vi "createPlatformData.vi"() -> (1 "platforms to \nlower":i32[](array[numeric]), 3 "platforms to \nraise":i32[](array[numeric]))   [LabVIEW 2017]
panel:
  in  "Platform 61":bool
  in  "Platform 60":bool
  in  "Platform 59":bool
  in  "Platform 58":bool
  in  "Platform 57":bool
  in  "Platform 56":bool
  in  "Platform 55":bool
  in  "Platform 54":bool
  in  "Platform 53":bool
  in  "Platform 52":bool
  in  "Platform 51":bool
  in  "Platform 50":bool
  in  "Platform 49":bool
  in  "Platform 48":bool
  in  "Platform 47":bool
  in  "Platform 46":bool
  in  "Platform 45":bool
  in  "Platform 44":bool
  in  "Platform 43":bool
  in  "Platform 42":bool
  in  "Platform 41":bool
  in  "Platform 40":bool
  in  "Platform 39":bool
  in  "Platform 38":bool
  in  "Platform 37":bool
  in  "Platform 36":bool
  in  "Platform 35":bool
  in  "Platform 34":bool
  in  "Platform 33":bool
  in  "Platform 32":bool
  in  "Platform 31":bool
  in  "Platform 30":bool
  in  "Platform 29":bool
  in  "Platform 28":bool
  in  "Platform 27":bool
  in  "Platform 26":bool
  in  "Platform 25":bool
  in  "Platform 24":bool
  in  "Platform 23":bool
  in  "Platform 22":bool
  in  "Platform 21":bool
  in  "Platform 20":bool
  in  "Platform 19":bool
  in  "Platform 18":bool
  in  "Platform 17":bool
  in  "Platform 16":bool
  in  "Platform 15":bool
  in  "Platform 14":bool
  in  "Platform 13":bool
  in  "Platform 12":bool
  in  "Platform 11":bool
  in  "Platform 10":bool
  in  "Platform 9":bool
  in  "Platform 8":bool
  in  "Platform 7":bool
  in  "Platform 6":bool
  in  "Platform 5":bool
  in  "Platform 4":bool
  in  "Platform 3":bool
  in  "Platform 2":bool
  in  "Platform 1":bool
  in  "Select?":bool
  in  "Platform 61":bool
  in  "Platform 60":bool
  in  "Platform 59":bool
  in  "Platform 58":bool
  in  "Platform 57":bool
  in  "Platform 56":bool
  in  "Platform 55":bool
  in  "Platform 54":bool
  in  "Platform 53":bool
  in  "Platform 52":bool
  in  "Platform 51":bool
  in  "Platform 50":bool
  in  "Platform 49":bool
  in  "Platform 48":bool
  in  "Platform 47":bool
  in  "Platform 46":bool
  in  "Platform 45":bool
  in  "Platform 44":bool
  in  "Platform 43":bool
  in  "Platform 42":bool
  in  "Platform 41":bool
  in  "Platform 40":bool
  in  "Platform 39":bool
  in  "Platform 38":bool
  in  "Platform 37":bool
  in  "Platform 36":bool
  in  "Platform 35":bool
  in  "Platform 34":bool
  in  "Platform 33":bool
  in  "Platform 32":bool
  in  "Platform 31":bool
  in  "Platform 30":bool
  in  "Platform 29":bool
  in  "Platform 28":bool
  in  "Platform 27":bool
  in  "Platform 26":bool
  in  "Platform 25":bool
  in  "Platform 24":bool
  in  "Platform 23":bool
  in  "Platform 22":bool
  in  "Platform 21":bool
  in  "Platform 20":bool
  in  "Platform 19":bool
  in  "Platform 18":bool
  in  "Platform 17":bool
  in  "Platform 16":bool
  in  "Platform 15":bool
  in  "Platform 14":bool
  in  "Platform 13":bool
  in  "Platform 12":bool
  in  "Platform 11":bool
  in  "Platform 10":bool
  in  "Platform 9":bool
  in  "Platform 8":bool
  in  "Platform 7":bool
  in  "Platform 6":bool
  in  "Platform 5":bool
  in  "Platform 4":bool
  in  "Platform 3":bool
  in  "Platform 2":bool
  in  "Platform 1":bool
  # "Platforms up"
  # "Platforms down"
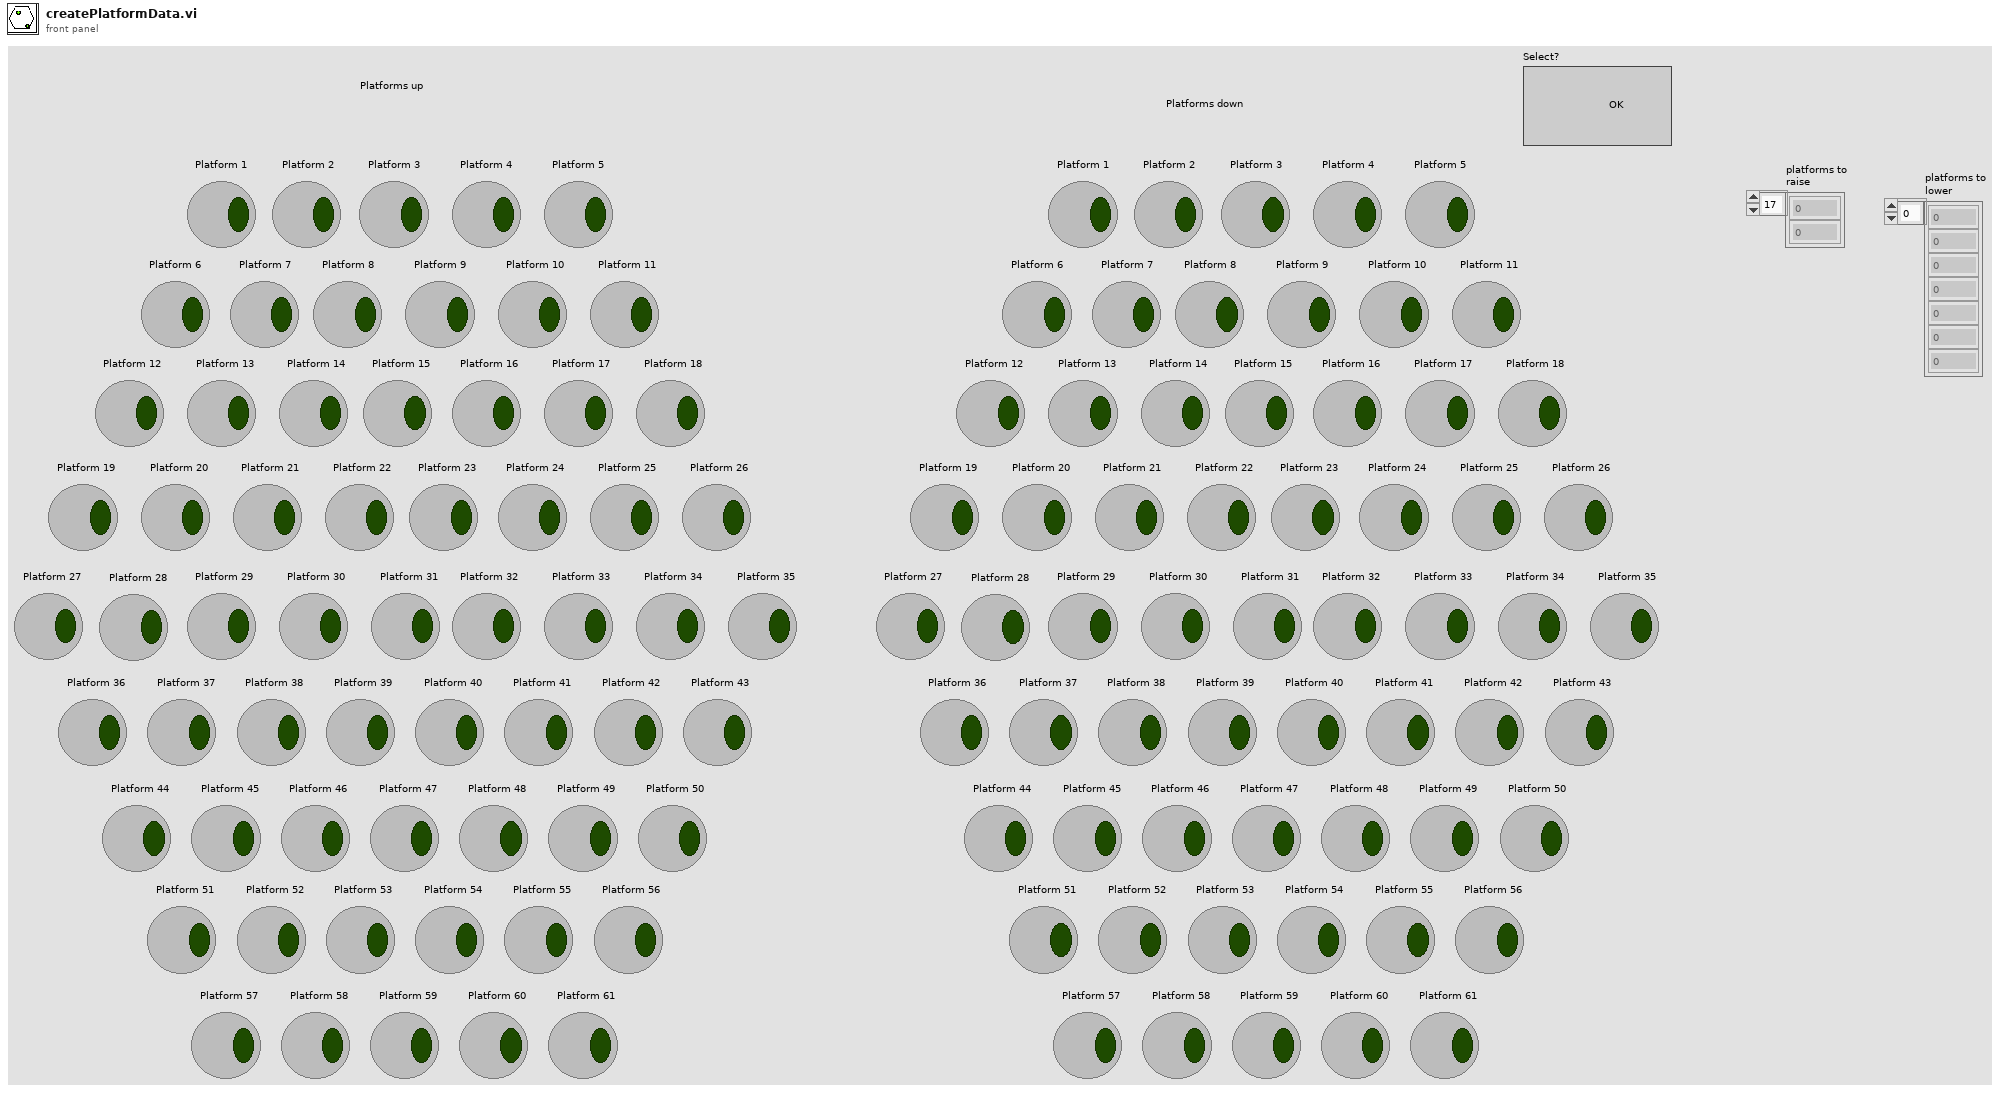
[diagram p1: front panel]
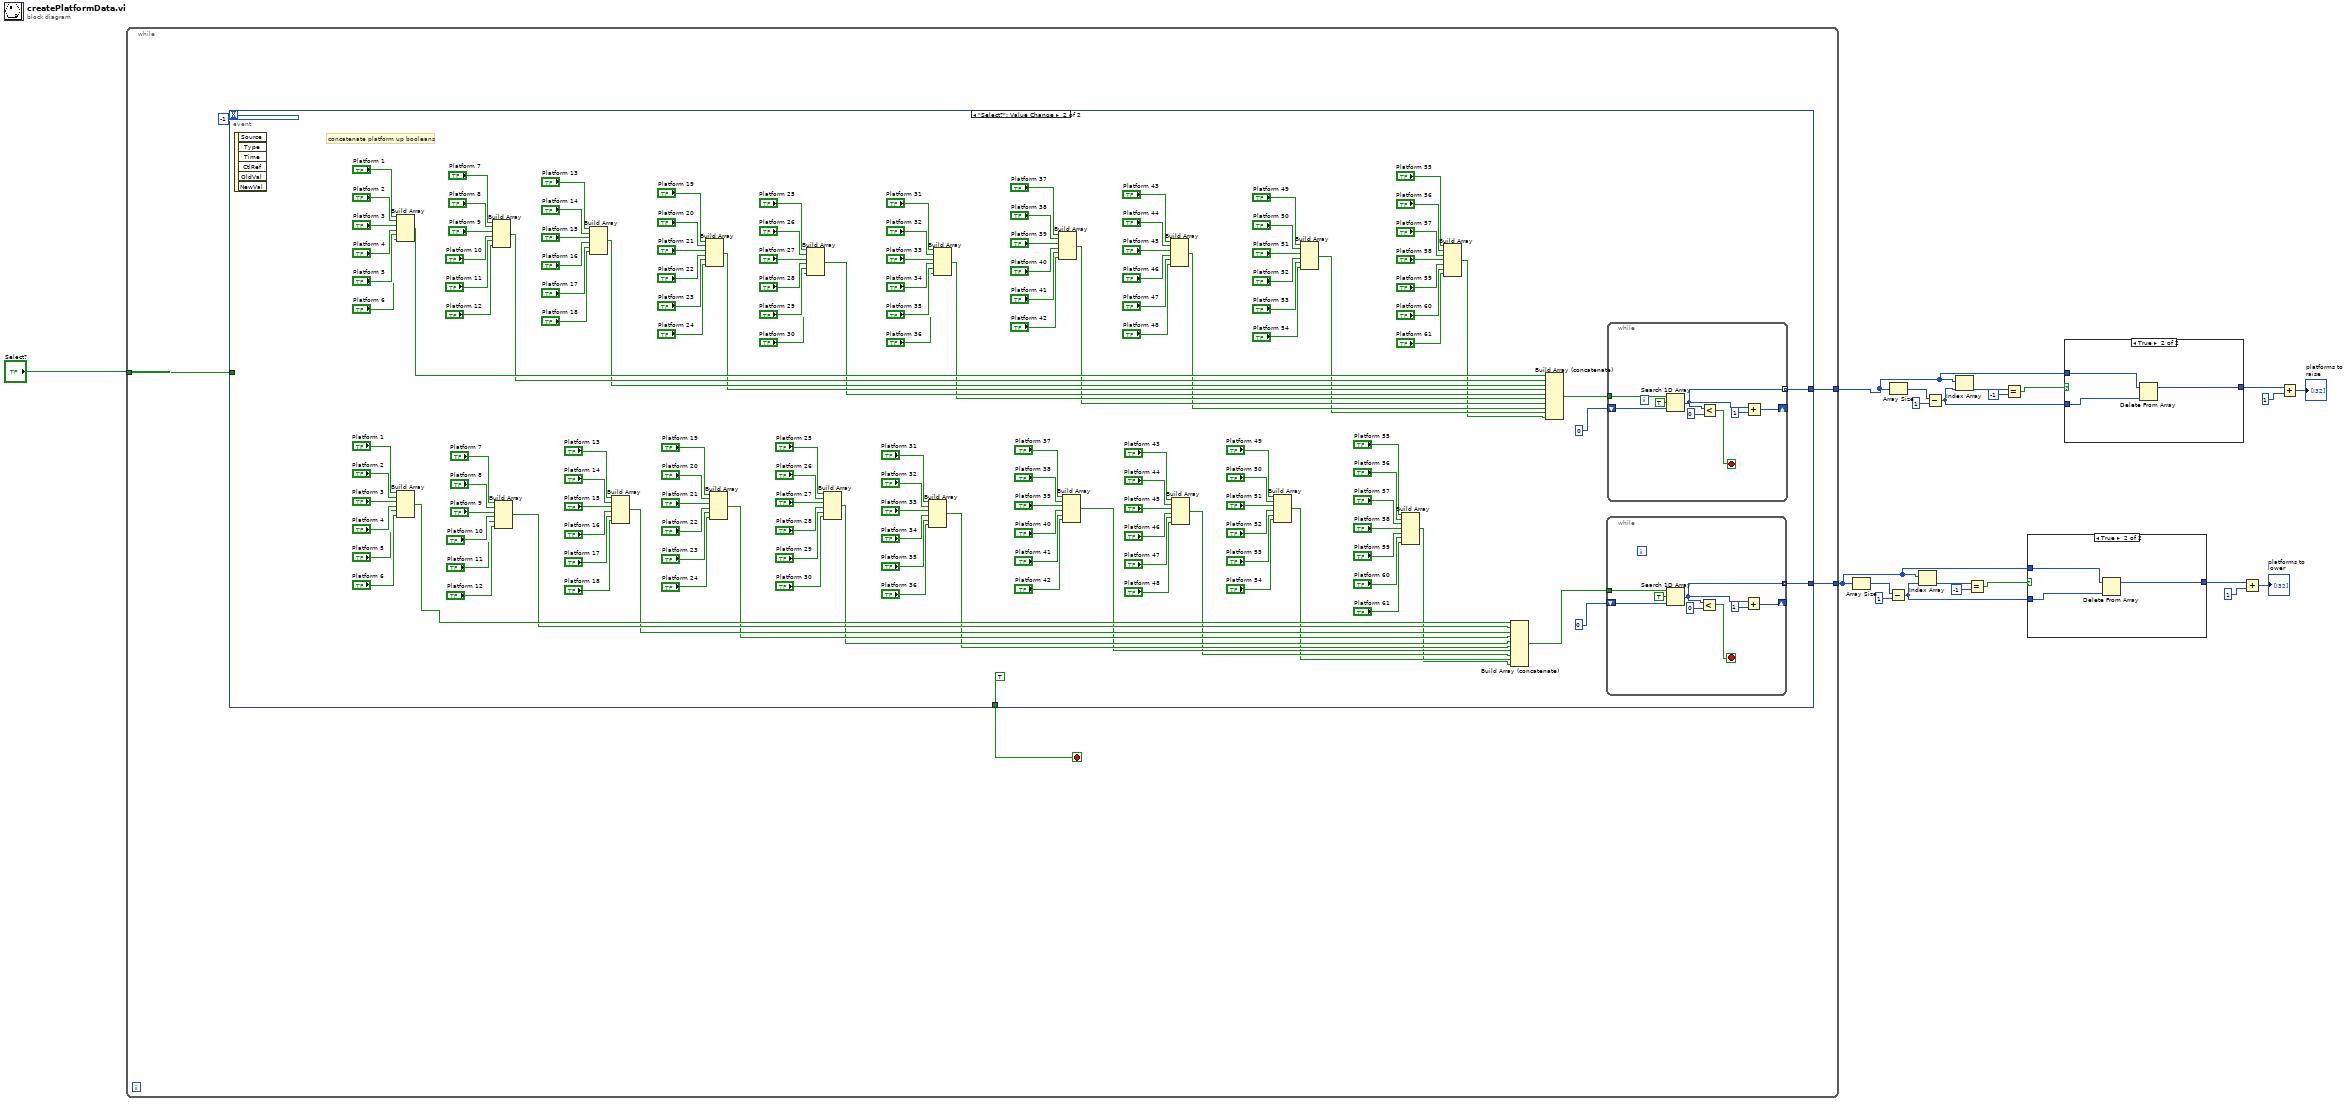
[diagram p0: block diagram]
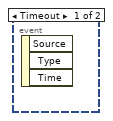
[diagram p4: hidden frame]
diagram:
  n1 = while {
    tunnel: "Select?" -> [w25]
    tunnel: [w23] -> w1
    tunnel: [w22] -> w17
    stop <- w24 stop-if-true
    n2 = event shown="[1] \"Select?\": Value Change" {
      selector: _ -> [_ _]
      dyn-events: _ -> [_ _]
      timeout: -1 -> [_ _]
      tunnel: w25 -> [_ _]
      tunnel: [_ TRUE] -> w24
      tunnel: [_ w41] -> w23
      tunnel: [_ w27] -> w22
      event Timeout {
        n3 = event-data() -> ()  [unwired: 1 in, 3 out]
      }
      event "Select?": Value Change {
        # "concatenate platform up booleans"
        n4 = event-data() -> ()  [unwired: 1 in, 6 out]
        n5 = Build Array("Platform 1", "Platform 2", "Platform 3", "Platform 4", "Platform 5", "Platform 6") -> (w39:bool[])
        n6 = Build Array("Platform 1", "Platform 2", "Platform 3", "Platform 4", "Platform 5", "Platform 6") -> (w53:bool[])
        n7 = Build Array("Platform 7", "Platform 8", "Platform 9", "Platform 10", "Platform 11", "Platform 12") -> (w52:bool[])
        n8 = Build Array("Platform 7", "Platform 8", "Platform 9", "Platform 10", "Platform 11", "Platform 12") -> (w38:bool[])
        n9 = Build Array("Platform 13", "Platform 14", "Platform 15", "Platform 16", "Platform 17", "Platform 18") -> (w51:bool[])
        n10 = Build Array("Platform 13", "Platform 14", "Platform 15", "Platform 16", "Platform 17", "Platform 18") -> (w37:bool[])
        n11 = Build Array("Platform 19", "Platform 20", "Platform 21", "Platform 22", "Platform 23", "Platform 24") -> (w50:bool[])
        n12 = Build Array("Platform 19", "Platform 20", "Platform 21", "Platform 22", "Platform 23", "Platform 24") -> (w36:bool[])
        n13 = Build Array("Platform 25", "Platform 26", "Platform 27", "Platform 28", "Platform 29", "Platform 30") -> (w49:bool[])
        n14 = Build Array("Platform 25", "Platform 26", "Platform 27", "Platform 28", "Platform 29", "Platform 30") -> (w35:bool[])
        n15 = Build Array("Platform 31", "Platform 32", "Platform 33", "Platform 34", "Platform 35", "Platform 36") -> (w34:bool[])
        n16 = Build Array("Platform 31", "Platform 32", "Platform 33", "Platform 34", "Platform 35", "Platform 36") -> (w48:bool[])
        n17 = Build Array("Platform 37", "Platform 38", "Platform 39", "Platform 40", "Platform 41", "Platform 42") -> (w47:bool[])
        n18 = Build Array("Platform 37", "Platform 38", "Platform 39", "Platform 40", "Platform 41", "Platform 42") -> (w33:bool[])
        n19 = Build Array("Platform 43", "Platform 44", "Platform 45", "Platform 46", "Platform 47", "Platform 48") -> (w46:bool[])
        n20 = Build Array("Platform 43", "Platform 44", "Platform 45", "Platform 46", "Platform 47", "Platform 48") -> (w32:bool[])
        n21 = Build Array("Platform 49", "Platform 50", "Platform 51", "Platform 52", "Platform 53", "Platform 54") -> (w31:bool[])
        n22 = Build Array("Platform 49", "Platform 50", "Platform 51", "Platform 52", "Platform 53", "Platform 54") -> (w45:bool[])
        n23 = Build Array("Platform 55", "Platform 56", "Platform 57", "Platform 58", "Platform 59", "Platform 60", "Platform 61") -> (w30:bool[])
        n24 = Build Array("Platform 55", "Platform 56", "Platform 57", "Platform 58", "Platform 59", "Platform 60", "Platform 61") -> (w44:bool[])
        n25 = Build Array (concatenate)(w39, w38, w37, w36, w35, w34, w33, w32, w31, w30) -> (w28:bool[])
        n26 = Build Array (concatenate)(w53, w52, w51, w50, w49, w48, w47, w46, w45, w44) -> (w43:bool[])
        n27 = while {
          tunnel: w28 -> [w176]
          shift-right: [w178] -> _
          shift-left: 0 ("start index (0)") -> [w182]
          tunnel: [w179] -> w27 mode=indexing
          stop <- w180 stop-if-true
          n28 = Search 1D Array(1D array=w176, element=TRUE, start index (0)=w182) -> (index of element=w179:i32)
          n29 = Less?(x=w179, y=0) -> (x < y?=w180:bool)
          n30 = Add(x=w179, y=1) -> (x+y=w178:i32)
        }
        n31 = while {
          tunnel: w43 -> [w191]
          shift-right: [w185] -> _
          shift-left: 0 ("start index (0)") -> [w189]
          tunnel: [w186] -> w41 mode=indexing
          stop <- w187 stop-if-true
          n32 = Search 1D Array(1D array=w191, element=TRUE, start index (0)=w189) -> (index of element=w186:i32)
          n33 = Less?(x=w186, y=0) -> (x < y?=w187:bool)
          n34 = Add(x=w186, y=1) -> (x+y=w185:i32)
        }
      }
    }
  }
  n35 = Array Size(array=w17) -> (size(s)=w15:i32)
  n36 = Subtract(x=w15, y=1) -> (x-y=w14:i32)
  n37 = Array Size(array=w1) -> (size(s)=w6:i32)
  n38 = Index Array(array=w17, index=w14) -> (element=w20:i32)
  n39 = Subtract(x=w6, y=1) -> (x-y=w5:i32)
  n40 = Index Array(array=w1, index=w5) -> (element=w10:i32)
  n41 = Equal?(x=w20, y=-1) -> (x = y?=w18:bool)
  n42 = Equal?(x=w10, y=-1) -> (x = y?=w8:bool)
  n43 = case shown="True" w18 {
    tunnel: w17 -> [w192 w195]
    tunnel: w14 -> [_ w194]
    tunnel: [w192 w193] -> w13
    frame False {
    }
    frame True {
      n44 = Delete From Array(array=w195, index=w194) -> (array with subset deleted=w193:i32[])  [unwired: 1 in, 1 out]
    }
  }
  n45 = case shown="True" w8 {
    tunnel: w1 -> [w196 w199]
    tunnel: w5 -> [_ w198]
    tunnel: [w196 w197] -> w4
    frame False {
    }
    frame True {
      n46 = Delete From Array(array=w199, index=w198) -> (array with subset deleted=w197:i32[])  [unwired: 1 in, 1 out]
    }
  }
  n47 = Add(x=w13, y=1) -> (x+y=→"platforms to \nlower":i32[])
  n48 = Add(x=w4, y=1) -> (x+y=→"platforms to \nraise":i32[])
